vi "Uneven Numeric Integration.vi"(10 "T":dbl[](array[numeric]), 11 "X":dbl[](array[numeric])) -> (0 "error":i32, 3 "result":dbl)   [LabVIEW 2017, in "NI_AALPro.lvlib"]
doc: "Performs numeric integration on the unevenly spaced values in the input array using the trapezoidal method."
uses:
  NI_AALPro.lvlib
  Real Dot Product.vi
  NI_AALBase.lvlib
panel:
  # "Uneven Numeric Integration"
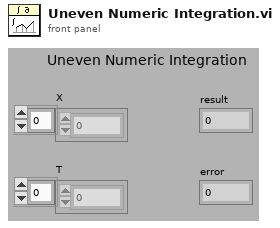
[diagram p1: front panel]
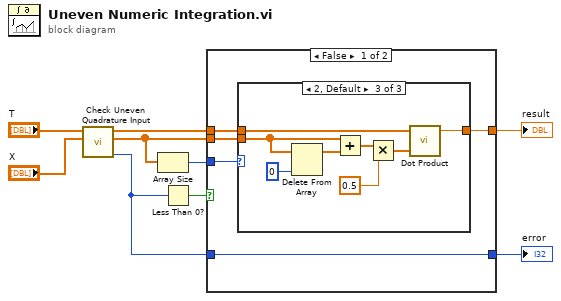
[diagram p0: block diagram]
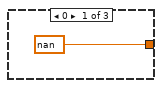
[diagram p2: hidden frame]
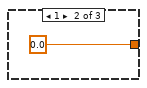
[diagram p3: hidden frame]
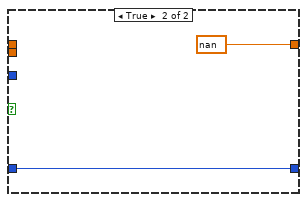
[diagram p4: hidden frame]
diagram:
  n1 = call "Check Uneven Quadrature Input.vi"("X In"="X", "T"="T") -> ("error"=w5:i32, "X Out"=w2:dbl[], "delta T"=w6:dbl[])  [unwired: 7 in]
  n2 = Array Size(array=w2) -> (size(s)=w1:i32)
  n3 = Less Than 0?(x=w5) -> (x < 0?=w7:bool)
  n4 = case shown="False" w7 {
    tunnel: w2 -> [w11 _]
    tunnel: w6 -> [w12 _]
    tunnel: w5 -> [w14 w26]
    tunnel: [w14 w26] -> w3
    tunnel: [w13 nan ("X * Y")] -> w4
    tunnel: w1 -> [w10 _]
    frame False {
      n5 = case shown="2, Default" w10 {
        tunnel: [nan 0.0 ("integration") w19] -> w13
        tunnel: w12 -> [_ _ w17]
        tunnel: w11 -> [_ _ w22]
        frame 0 {
        }
        frame 1 {
        }
        frame 2, Default {
          n6 = Delete From Array(array=w22, index=0) -> (array with subset deleted=w23:dbl[])  [unwired: 1 in, 1 out]
          n7 = Add(x=w22, y=w23) -> (x+y=w21:dbl[])
          n8 = Multiply(x=w21, y=0.5) -> (x*y=w18:dbl[])
          n9 = call-poly "Dot Product.vi"("Y Vector"=w18, "X Vector"=w17) -> ("X * Y"=w19:dbl)  [unwired: 1 out]
        }
      }
    }
    frame True {
    }
  }
  "result" <- w4
  "error" <- w3
